vi "Begin.vi"(8 "error in":errorcluster) -> (0 "error out":errorcluster)   [LabVIEW 2016]
doc: "Called before other user functions, this VI is expected to open initial I/O refnums, load in file data, and do all program initialization. Notice that the <B>error out</B> terminal is simply used for data flow. Wiring it to other structures or subVIs ensures that this VI runs first."
uses:
  <vilib>/Rock Robotics/WPI/DriverStation/WPI_DriverStationRobotMode2.ctl
  <vilib>/Rock Robotics/WPI/Joystick/WPI_JoystickDeviceEnum.ctl
  <vilib>/Rock Robotics/WPI/ThirdParty/CanMotor/TalonSRX/WPI_CANTalonSRX_APIControlMode.ctl
  <vilib>/Rock Robotics/WPI/ThirdParty/CanMotor/TalonSRX/WPI_CANTalonSRX_APIFeedbackSelect.ctl
  <vilib>/Rock Robotics/SystemInterfaces/DIO/FPGA_DIOChannel.ctl
  <vilib>/Rock Robotics/SystemInterfaces/spilib/spi_bus.ctl
  <vilib>/Rock Robotics/SystemInterfaces/DIO/FPGA_DIOPWMChannel.ctl
  <vilib>/Rock Robotics/WPI/SafetyOutput/WPI_SafetyOutputConfigMenu.ctl
  Robot Global Data.vi
  <vilib>/Rock Robotics/Network Tables/NT Write String Array.vi
  <vilib>/Rock Robotics/WPI/Counter/WPI_CounterDigitalInputToDigitalSource.vi
  <vilib>/Rock Robotics/WPI/Switch/WPI_SwitchOpenLimit.vi
  <vilib>/Rock Robotics/WPI/Gyro/WPI_GyroAnalogOpen.vi
  <vilib>/Rock Robotics/WPI/RobotDrive/WPI_RobotDriveOpen4MotorWithExistingMotors.vi
  <vilib>/Rock Robotics/WPI/RobotDrive/WPI_RobotDriveOpen4MotorWithTalon.vi
  <vilib>/Rock Robotics/WPI/MotorControl/WPI_MotorControlOpen SPARK.vi
  <vilib>/Rock Robotics/WPI/MotorControl/WPI_MotorControlOpen Victor.vi
  <vilib>/Rock Robotics/WPI/Solenoid/WPI_SolenoidOpenSingle.vi
  <vilib>/Rock Robotics/WPI/Solenoid/WPI_SolenoidChannel.ctl
panel:
  out "error out 2":errorcluster
  in  "Number Encoder Lines\n(Counts Per Rotation)":u32=309
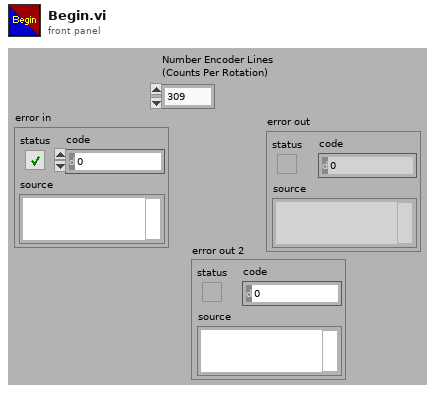
[diagram p1: front panel]
types:
  T1 = typedef "spi_bus.ctl" = enum16{"SPI On-Board, CS0", "SPI On-Board, CS1", "SPI On-Board, CS2", "SPI On-Board, CS3", "SPI MXP", "Invalid"}
  T2 = typedef "FPGA_DIOChannel.ctl" = enum8{"DIO 0", "DIO 1", "DIO 2", "DIO 3", "DIO 4", "DIO 5", "DIO 6", "DIO 7", "DIO 8", "DIO 9", "DIO MXP 0", "DIO MXP 1", "DIO MXP 2", "DIO MXP 3", "DIO MXP 4", "DIO MXP 5", "DIO MXP 6", "DIO MXP 7", "DIO MXP 8", "DIO MXP 9", "DIO MXP 10", "DIO MXP 11", "DIO MXP 12", "DIO MXP 13", "DIO MXP 14", "DIO MXP 15", "SPI Port CS1", "SPI Port CS2", "SPI Port CS3", "SPI Port MISO", "SPI Port MOSI", "Invalid"}
  T3 = typedef "WPI_CANTalonSRX_APIFeedbackSelect.ctl" = enum16{"Digital Quadrature Encoder", "Analog Potentiometer", "Analog Encoder", "Count on Quad-A (Rising-Edge)", "Count on Quad-A (Falling-Edge)", "CTR Magnetic Enc (Absolute)", "CTR Magnetic Enc (Relative)", "Pulse Width"}
  T4 = typedef "WPI_CANTalonSRX_APIControlMode.ctl" = enum8{"Percent VBus", "Speed", "Position", "Slave", "Unchanged / Invalid", "Voltage Compensation", "Current", "Motion Profile", "Motion Magic"}
  T5 = typedef "WPI_JoystickDeviceEnum.ctl" = enum16{"USB 0", "USB 1", "USB 2", "USB 3", "USB 4", "USB 5"}
  T6 = typedef "WPI_DriverStationRobotMode2.ctl" = enum16{"Autonomous Disabled", "Autonomous Enabled", "Teleop Disabled", "Teleop Enabled", "Disconnected", "Finish", "Test Disabled", "Test Enabled", "Emergency Stopped"}
  T7 = typedef "WPI_MotorControlDeviceRef.ctl" = cluster{"DeviceStatus":errorcluster, "Type":T8, "PWM":cluster{"PWM Channel":T9, "DeadBand":T10}, "CAN":cluster{"Device Number":u8, "SetOutput VI Ref":variant, "GetOutput VI Ref":variant, "Enable VI Ref":variant, "Disable VI Ref":variant, "Data":variant}, "Invert":bool}
  T8 = typedef "WPI_MotorControlType.ctl" = enum16{"PWM", "CAN"}
  T9 = typedef "FPGA_DIOPWMChannel.ctl" = enum8{"PWM 0", "PWM 1", "PWM 2", "PWM 3", "PWM 4", "PWM 5", "PWM 6", "PWM 7", "PWM 8", "PWM 9", "PWM MXP 0", "PWM MXP 1", "PWM MXP 2", "PWM MXP 3", "PWM MXP 4", "PWM MXP 5", "PWM MXP 6", "PWM MXP 7", "PWM MXP 8", "PWM MXP 9", "Invalid"}
  T10 = typedef "WPI_PWMDeadband.ctl" = cluster{"Name":string, "maxPositivePwm":i32, "minPositivePwm":i32, "centerPwm":i32, "maxNegativePwm":i32, "minNegativePwm":i32, "angularRange":u16}
  T11 = typedef "WPI_GyroDevRef.ctl" = cluster{"DevStatus":errorcluster, "Analog Channel":T12, "Offset":dbl, "Gain (VoltsPerDegree/Second)":dbl, "Gyro Type":enum16{"Analog", "XRS450"}, "Handle":i32, "SPI Bus":T1, "Device Found":bool, "Sample Rate":dbl, "Calibrate On Open":bool}
  T12 = typedef "FPGA_AIChannel.ctl" = enum8{"AI 0", "AI 1", "AI 2", "AI 3", "AI MXP 0", "AI MXP 1", "AI MXP 2", "AI MXP 3", "Invalid"}
  T13 = typedef "WPI_SafetyOutputConfigMenu.ctl" = enum16{"Enable", "Disable"}
  T14 = typedef "WPI_RobotDriveDevRef.ctl" = cluster{"DevStatus":errorcluster, "Motors[]":T7[], "Square Inputs":bool, "Max Output":dbl}
  T15 = typedef "WPI_ServoDeviceRef.ctl" = cluster{"DeviceStatus":errorcluster, "PWM Channel":T9, "DeadBand":T10}
  T16 = typedef "WPI_JoystickDevRef.ctl" = cluster{"Device":T5}
  T17 = typedef "WPI_SwitchDevRef.ctl" = cluster{"DevStatus":errorcluster, "DIO Channel":T2, "CntIndex":T18, "Normally Closed":bool}
  T18 = typedef "FPGA_CounterCtrSystemIndex.ctl" = enum8{"Ctr 0", "Ctr 1", "Ctr 2", "Ctr 3", "Ctr 4", "Ctr 5", "Ctr 6", "Ctr 7", "Invalid"}
  T19 = typedef "WPI_SolenoidChannel.ctl" = enum8{"Solenoid 0", "Solenoid 1", "Solenoid 2", "Solenoid 3", "Solenoid 4", "Solenoid 5", "Solenoid 6", "Solenoid 7", "Invalid"}
  T20 = typedef "WPI_SolenoidDevRef.ctl" = cluster{"DevStatus":errorcluster, "Pneumatics Control Module":u8, "Forward Solenoid Channel":T19, "Reverse Solenoid Channel":T19}
  T21 = typedef "WPI_DigitalInputDevRef.ctl" = cluster{"DevStatus":errorcluster, "DIO Channel":T2}
  T22 = typedef "FPGA_CounterEncoderSourceConvertionLVSourceType.ctl" = cluster{"DevStatus":errorcluster, "AnalogTriggerMode?":bool, "DigitalMode":cluster{"DIO Channel":T23}, "AnalogTriggerMode":cluster{"AnalogTriggerIndex":T24, "OutputType":T25}}
  T23 = typedef "FPGA_DIODigitalSourceChannel.ctl" = enum8{"DIO 0", "DIO 1", "DIO 2", "DIO 3", "DIO 4", "DIO 5", "DIO 6", "DIO 7", "DIO 8", "DIO 9", "DIO MXP 0", "DIO MXP 1", "DIO MXP 2", "DIO MXP 3", "DIO MXP 4", "DIO MXP 5", "DIO MXP 6", "DIO MXP 7", "DIO MXP 8", "DIO MXP 9", "DIO MXP 10", "DIO MXP 11", "DIO MXP 12", "DIO MXP 13", "DIO MXP 14", "DIO MXP 15", "Disabled"}
  T24 = typedef "FPGA_AnalogTriggerIndex.ctl" = enum8{"Trig 0", "Trig 1", "Trig 2", "Trig 3", "Trig 4", "Trig 5", "Trig 6", "Trig 7", "Invalid"}
  T25 = typedef "FPGA_AnalogTriggerOutType.ctl" = enum16{"InWindow", "TriggerState", "Rising", "Falling"}
  T26 = typedef "WPI_EncoderDevRef.ctl" = cluster{"DevStatus":errorcluster, "EncoderIndex":T27, "CounterIndex":T18, "DistancePerCount":dbl, "Decoding Type":T28}
  T27 = typedef "FPGA_EncoderIdx.ctl" = enum8{"Enc 0", "Enc 1", "Enc 2", "Enc 3", "Enc 4", "Enc 5", "Enc 6", "Enc 7", "Invalid"}
  T28 = typedef "WPI_EncoderType.ctl" = enum16{"1x", "2x", "4x"}
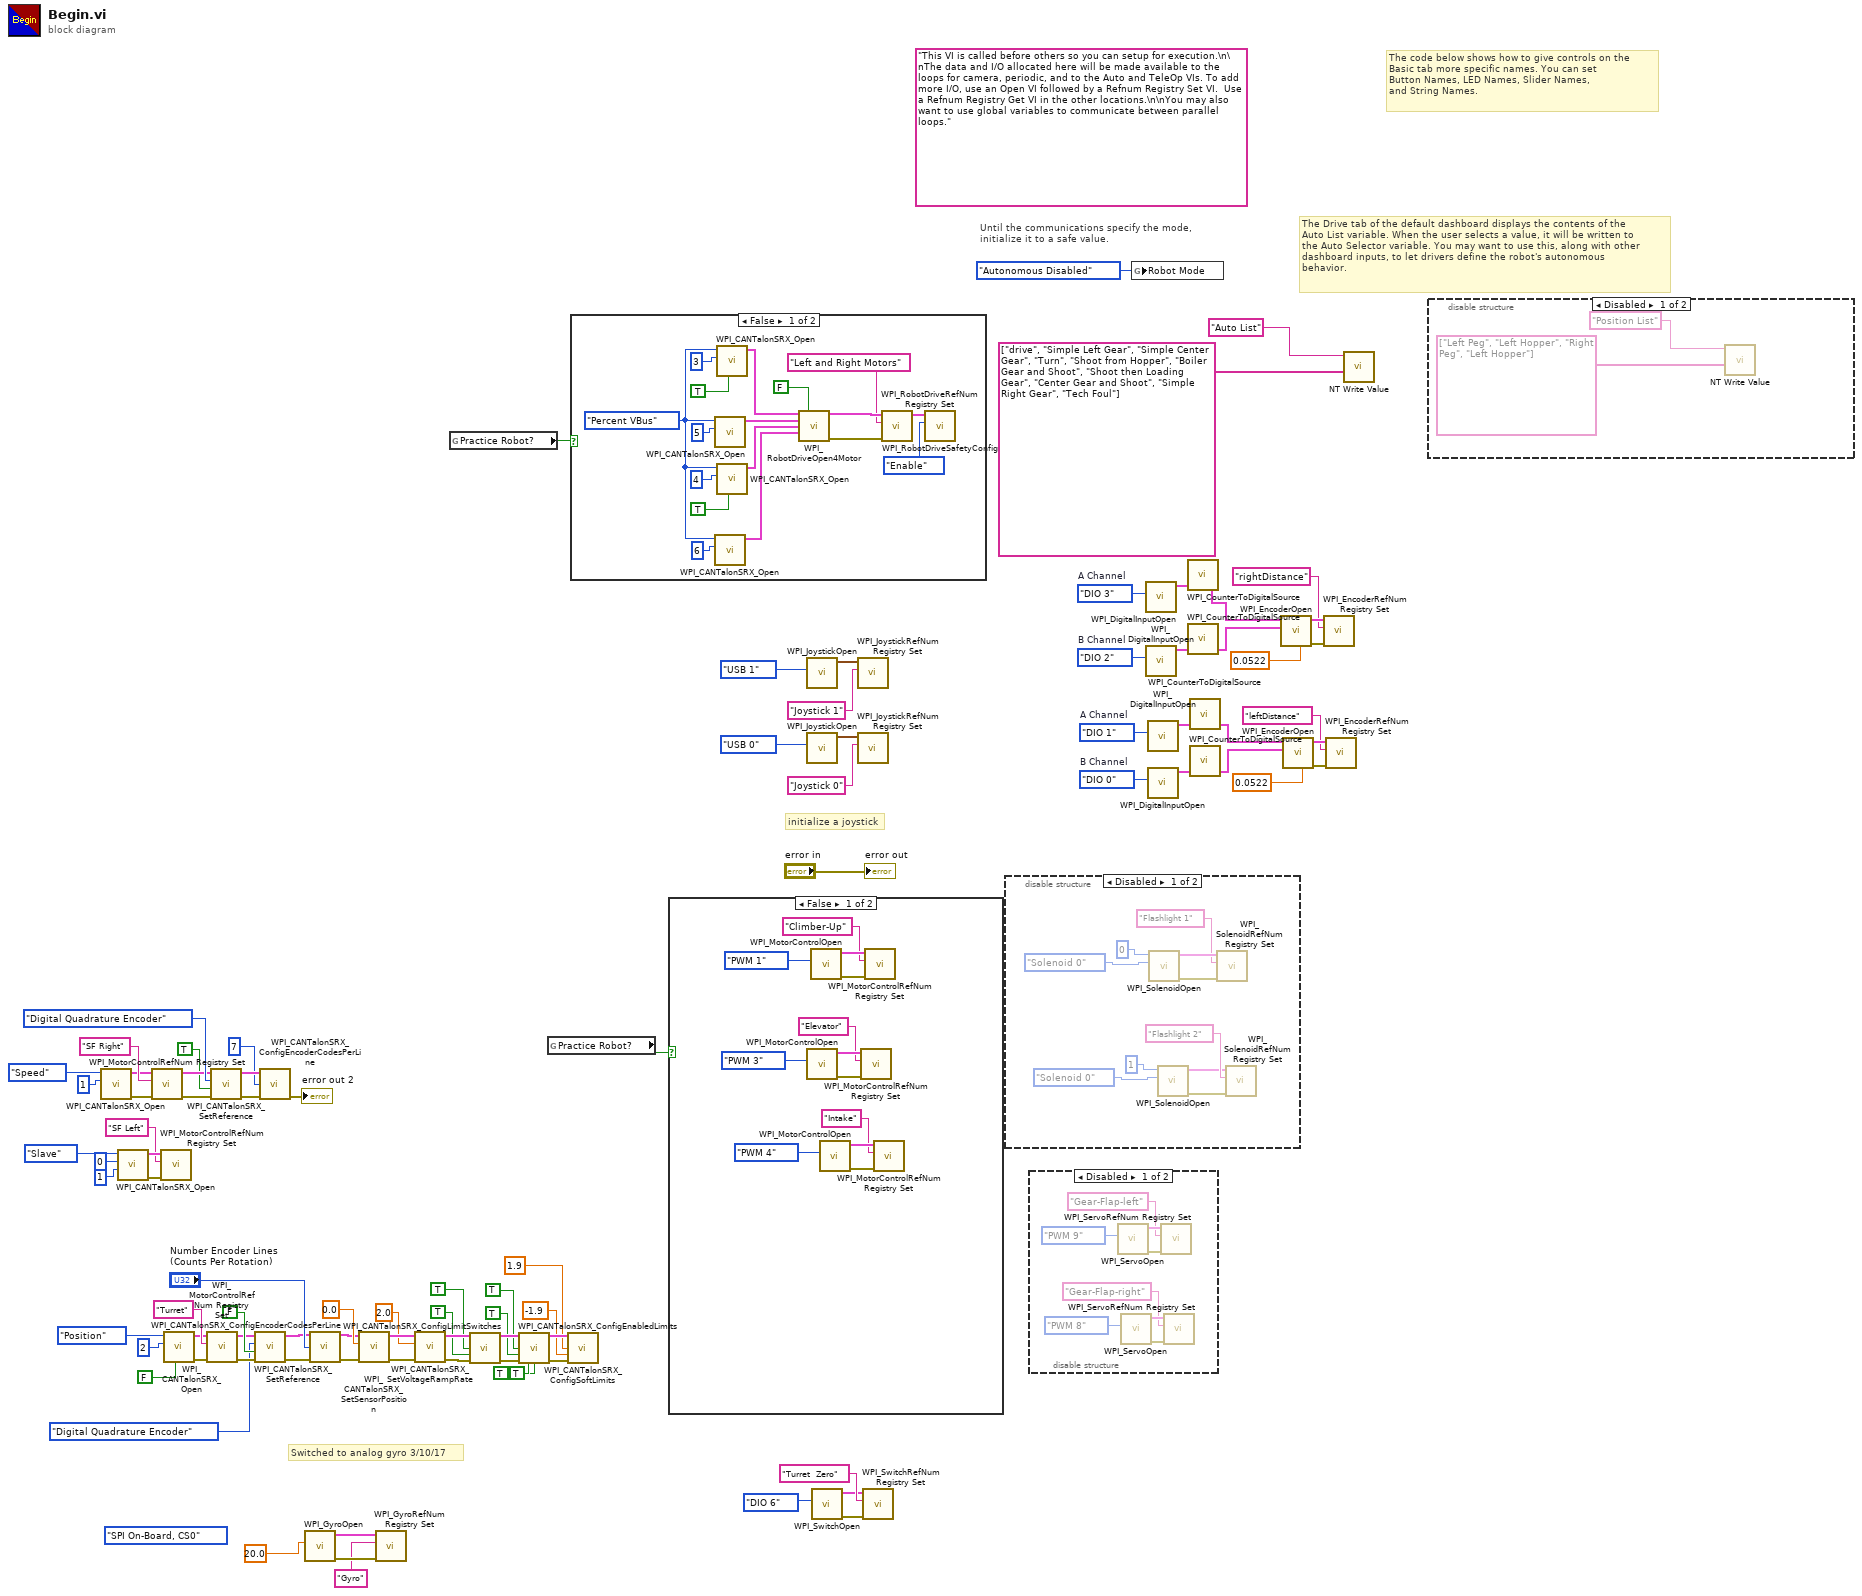
[diagram p0: block diagram]
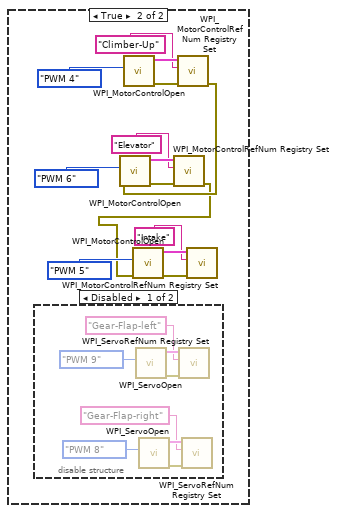
[diagram p5: hidden frame]
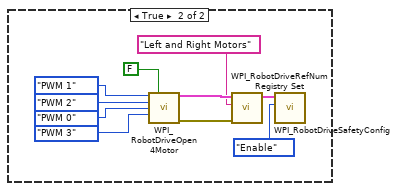
[diagram p7: hidden frame]
diagram:
  (unwired) spi_bus."SPI On-Board, CS0" ("SPI Bus")
  w38 = FPGA_DIOChannel."DIO 2"  # B Channel
  w37 = FPGA_DIOChannel."DIO 3"  # A Channel
  w47 = FPGA_DIOChannel."DIO 0"  # B Channel
  w46 = FPGA_DIOChannel."DIO 1"  # A Channel
  (unwired) "This VI is called before others so you can setup for execution.\n\nThe data and I/O allocated here will be made available to the loops for camera, periodic, and to the Auto and TeleOp VIs. To add more I/O, use an Open VI followed by a Refnum Registry Set VI.  Use a Refnum Registry Get VI in the other locations.\n\nYou may also want to use global variables to communicate between parallel loops."
  # "Switched to analog gyro 3/10/17"
  # "The Drive tab of the default dashboard displays the contents of the\nAuto List variable. When the user selects a value, it will be written to\nthe Auto Selector variable. You may want to use this, along with other\ndashboard inputs, to let drivers define the robot's autonomous\nbehavior."
  # "The code below shows how to give controls on the\nBasic tab more specific names. You can set\nButton Names, LED Names, Slider Names,\nand String Names."
  # "initialize a joystick"
  # "Until the communications specify the mode,\ninitialize it to a safe value."
  n1 = call <vilib>:"WPI_CANTalonSRX_Open.vi"("Device Number"=u8 1, "Control Mode"=WPI_CANTalonSRX_APIControlMode."Speed") -> ("error out"=w68:errorcluster, "CAN Talon SRX Ref"=w67:T7)  [unwired: 8 in]
  n2 = call <vilib>:"WPI_CANTalonSRX_Open.vi"("Master Device Number"=u8 1, "Device Number"=u8 0, "Control Mode"=WPI_CANTalonSRX_APIControlMode."Slave") -> ("error out"=w75:errorcluster, "CAN Talon SRX Ref"=w76:T7)  [unwired: 7 in]
  n3 = call <vilib>:"WPI_MotorControlRefNum Registry Set.vi"("error in (no error)"=w68, "refnum name"="SF Right", "MotorControlDevRef"=w67) -> ("error out"=w49:errorcluster, "MotorControlDevRef"=w50:T7)  [unwired: 7 in]
  n4 = call <vilib>:"WPI_MotorControlRefNum Registry Set.vi"("error in (no error)"=w75, "refnum name"="SF Left", "MotorControlDevRef"=w76) -> ()  [unwired: 7 in, 2 out]
  n5 = call <vilib>:"WPI_CANTalonSRX_Open.vi"("Invert"=FALSE, "Device Number"=u8 2, "Control Mode"=WPI_CANTalonSRX_APIControlMode."Position") -> ("error out"=w59:errorcluster, "CAN Talon SRX Ref"=w61:T7)  [unwired: 7 in]
  n6 = call <vilib>:"WPI_MotorControlRefNum Registry Set.vi"("error in (no error)"=w59, "refnum name"="Turret", "MotorControlDevRef"=w61) -> ("error out"=w58:errorcluster, "MotorControlDevRef"=w60:T7)  [unwired: 7 in]
  n7 = call <vilib>:"WPI_CANTalonSRX_SetReference.vi"("error in (no error)"=w49, "Reverse Feedback Sensor"=TRUE, "Feedback Reference"=WPI_CANTalonSRX_APIFeedbackSelect."Digital Quadrature Encoder", "CAN Talon SRX Ref"=w50) -> ("error out"=w48:errorcluster, "CAN Talon SRX Ref"=w53:T7)  [unwired: 6 in]
  n8 = call <vilib>:"WPI_CANTalonSRX_SetReference.vi"("error in (no error)"=w58, "Reverse Feedback Sensor"=FALSE, "Feedback Reference"=WPI_CANTalonSRX_APIFeedbackSelect."Digital Quadrature Encoder", "CAN Talon SRX Ref"=w60) -> ("error out"=w57:errorcluster, "CAN Talon SRX Ref"=w63:T7)  [unwired: 6 in]
  n9 = call <vilib>:"WPI_CANTalonSRX_ConfigEncoderCodesPerLine.vi"("CAN Talon SRX Ref"=w53, "Number Encoder Lines\n(Counts Per Rotation)"=u32 7 ("Number Encoder Lines\n(Counts Per Rotation)"), "error in (no error)"=w48) -> ("error out"=→"error out 2":errorcluster)  [unwired: 11 in, 1 out]
  n10 = call-poly <vilib>:"WPI_GyroOpen.vi"("Analog Channel"=20.0 ("Calibration Time (s)")) -> ("error out"=w20:errorcluster, "GyroDevRef"=w19:T11)  [unwired: 8 in, 1 out]
  n11 = call <vilib>:"WPI_CANTalonSRX_ConfigEncoderCodesPerLine.vi"("CAN Talon SRX Ref"=w63, "Number Encoder Lines\n(Counts Per Rotation)"="Number Encoder Lines\n(Counts Per Rotation)", "error in (no error)"=w57) -> ("CAN Talon SRX Ref"=w55:T7, "error out"=w56:errorcluster)  [unwired: 11 in]
  n12 = call <vilib>:"WPI_CANTalonSRX_SetSensorPosition.vi"("error in (no error)"=w56, "New Sensor Position"=0.0, "CAN Talon SRX Ref"=w55) -> ("error out"=w23:errorcluster, "CAN Talon SRX Ref"=w22:T7)  [unwired: 7 in]
  n13 = call <vilib>:"WPI_GyroRefNum Registry Set.vi"("error in (no error)"=w20, "refnum name"="Gyro", "GyroDevRef"=w19) -> ()  [unwired: 7 in, 2 out]
  n14 = call <vilib>:"WPI_CANTalonSRX_SetVoltageRampRate.vi"("error in (no error)"=w23, "Throttle Ramp Rate (percent/s)"=2.0, "CAN Talon SRX Ref"=w22) -> ("error out"=w13:errorcluster, "CAN Talon SRX Ref"=w14:T7)  [unwired: 7 in]
  n15 = global read "Robot Global Data.vi" "Practice Robot?"() -> (w82:bool)
  n16 = call <vilib>:"WPI_CANTalonSRX_ConfigLimitSwitches.vi"("CAN Talon SRX Ref"=w14, "Forward Limit Switch Normally Open"=TRUE, "Reverse Limit Switch Normally Open"=TRUE, "error in (no error)"=w13) -> ("CAN Talon SRX Ref"=w10:T7, "error out"=w9:errorcluster)  [unwired: 10 in]
  n17 = call <vilib>:"WPI_CANTalonSRX_ConfigEnabledLimits.vi"("CAN Talon SRX Ref"=w10, "Forward Limit Switch Enable"=TRUE, "Reverse Limit Switch Enable"=TRUE, "error in (no error)"=w9, "Forward Soft Limit Enable"=TRUE, "Reverse Soft Limit Enable"=TRUE) -> ("CAN Talon SRX Ref"=w6:T7, "error out"=w5:errorcluster)  [unwired: 8 in]
  n18 = global read "Robot Global Data.vi" "Practice Robot?"() -> (w81:bool)
  n19 = call <vilib>:"WPI_CANTalonSRX_ConfigSoftLimits.vi"("CAN Talon SRX Ref"=w6, "Forward Limit Position"=1.9 ("Upper Limit Position"), "Reverse Limit Position"=-1.9 ("Lower Limit Position"), "error in (no error)"=w5) -> ()  [unwired: 10 in, 2 out]
  n20 = case shown="False" w82 {
    frame False {
      w100 = WPI_CANTalonSRX_APIControlMode."Percent VBus" ("Control Mode")
      n21 = call <vilib>:"WPI_CANTalonSRX_Open.vi"("Device Number"=u8 5, "Control Mode"=w100) -> ("CAN Talon SRX Ref"=w103:T7)  [unwired: 8 in, 1 out]
      n22 = call <vilib>:"WPI_CANTalonSRX_Open.vi"("Device Number"=u8 6, "Control Mode"=w100) -> ("CAN Talon SRX Ref"=w101:T7)  [unwired: 8 in, 1 out]
      n23 = call <vilib>:"WPI_CANTalonSRX_Open.vi"("Invert"=TRUE, "Device Number"=u8 3, "Control Mode"=w100) -> ("CAN Talon SRX Ref"=w104:T7)  [unwired: 7 in, 1 out]
      n24 = call <vilib>:"WPI_CANTalonSRX_Open.vi"("Invert"=TRUE, "Device Number"=u8 4, "Control Mode"=w100) -> ("CAN Talon SRX Ref"=w102:T7)  [unwired: 7 in, 1 out]
      n25 = call-poly <vilib>:"WPI_RobotDriveOpen4Motor.vi"("Rear Left Motor Dev Ref"=w104, "Square Inputs"=FALSE, "Rear Right Motor Dev Ref"=w103, "Front Left Motor Dev Ref"=w102, "Front Right Motor Dev Ref"=w101) -> ("RobotDriveDevRef"=w109:T14, "error out"=w107:errorcluster)  [unwired: 9 in]
      n26 = call <vilib>:"WPI_RobotDriveRefNum Registry Set.vi"("error in (no error)"=w107, "refnum name"="Left and Right Motors", "RobotDriveDevRef"=w109) -> ("RobotDriveDevRef"=w106:T14)  [unwired: 1 in, 7 out]
      n27 = call <vilib>:"WPI_RobotDriveSafetyConfig.vi"("mode"=WPI_SafetyOutputConfigMenu."Enable", "RobotDriveDevRef"=w106) -> ()  [unwired: 8 in, 2 out]
    }
    frame True {
      n28 = call-poly <vilib>:"WPI_RobotDriveOpen4Motor.vi"("Rear Left Motor"=FPGA_DIOPWMChannel."PWM 1", "Rear Left Motor Inverted"=FALSE ("Square Inputs"), "Rear Right Motor"=FPGA_DIOPWMChannel."PWM 2", "Front Left Motor"=FPGA_DIOPWMChannel."PWM 0", "Front Right Motor"=FPGA_DIOPWMChannel."PWM 3") -> ("RobotDriveDevRef"=w119:T14, "error out"=w117:errorcluster)  [unwired: 9 in]
      n29 = call <vilib>:"WPI_RobotDriveRefNum Registry Set.vi"("error in (no error)"=w117, "refnum name"="Left and Right Motors", "RobotDriveDevRef"=w119) -> ("RobotDriveDevRef"=w116:T14)  [unwired: 1 in, 7 out]
      n30 = call <vilib>:"WPI_RobotDriveSafetyConfig.vi"("mode"=WPI_SafetyOutputConfigMenu."Enable", "RobotDriveDevRef"=w116) -> ()  [unwired: 8 in, 2 out]
    }
  }
  n31 = case shown="False" w81 {
    frame False {
      n32 = call-poly <vilib>:"WPI_MotorControlOpen.vi"("PWM Channel"=FPGA_DIOPWMChannel."PWM 3") -> ("error out"=w131:errorcluster, "MotorControlDeviceRef"=w130:T7)  [unwired: 9 in]
      n33 = call-poly <vilib>:"WPI_MotorControlOpen.vi"("PWM Channel"=FPGA_DIOPWMChannel."PWM 1") -> ("error out"=w127:errorcluster, "MotorControlDeviceRef"=w126:T7)  [unwired: 9 in]
      n34 = call-poly <vilib>:"WPI_MotorControlOpen.vi"("PWM Channel"=FPGA_DIOPWMChannel."PWM 4") -> ("error out"=w123:errorcluster, "MotorControlDeviceRef"=w122:T7)  [unwired: 9 in]
      n35 = call <vilib>:"WPI_MotorControlRefNum Registry Set.vi"("error in (no error)"=w131, "refnum name"="Elevator", "MotorControlDevRef"=w130) -> ()  [unwired: 7 in, 2 out]
      n36 = call <vilib>:"WPI_MotorControlRefNum Registry Set.vi"("error in (no error)"=w127, "refnum name"="Climber-Up", "MotorControlDevRef"=w126) -> ()  [unwired: 7 in, 2 out]
      n37 = call <vilib>:"WPI_MotorControlRefNum Registry Set.vi"("error in (no error)"=w123, "refnum name"="Intake", "MotorControlDevRef"=w122) -> ()  [unwired: 7 in, 2 out]
    }
    frame True {
      n38 = disable-structure shown="Disabled" {
        frame Disabled {
          n39 = call <vilib>:"WPI_ServoOpen.vi"("PWM Channel"=FPGA_DIOPWMChannel."PWM 9") -> ("error out"=w148:errorcluster, "ServoDeviceRef"=w153:T15)  [unwired: 9 in]
          n40 = call <vilib>:"WPI_ServoOpen.vi"("PWM Channel"=FPGA_DIOPWMChannel."PWM 8") -> ("error out"=w149:errorcluster, "ServoDeviceRef"=w152:T15)  [unwired: 9 in]
          n41 = call <vilib>:"WPI_ServoRefNum Registry Set.vi"("error in (no error)"=w148, "refnum name"="Gear-Flap-left", "ServoDeviceRef"=w153) -> ()  [unwired: 7 in, 2 out]
          n42 = call <vilib>:"WPI_ServoRefNum Registry Set.vi"("error in (no error)"=w149, "refnum name"="Gear-Flap-right", "ServoDeviceRef"=w152) -> ()  [unwired: 7 in, 2 out]
        }
        frame Enabled {
        }
      }
      n43 = call-poly <vilib>:"WPI_MotorControlOpen.vi"("PWM Channel"=FPGA_DIOPWMChannel."PWM 4") -> ("error out"=w141:errorcluster, "MotorControlDeviceRef"=w140:T7)  [unwired: 9 in]
      n44 = call <vilib>:"WPI_MotorControlRefNum Registry Set.vi"("error in (no error)"=w141, "refnum name"="Climber-Up", "MotorControlDevRef"=w140) -> ("error out"=w133:errorcluster)  [unwired: 7 in, 1 out]
      n45 = call-poly <vilib>:"WPI_MotorControlOpen.vi"("error in (no error)"=w133, "PWM Channel"=FPGA_DIOPWMChannel."PWM 6") -> ("error out"=w145:errorcluster, "MotorControlDeviceRef"=w144:T7)  [unwired: 8 in]
      n46 = call <vilib>:"WPI_MotorControlRefNum Registry Set.vi"("error in (no error)"=w145, "refnum name"="Elevator", "MotorControlDevRef"=w144) -> ("error out"=w132:errorcluster)  [unwired: 7 in, 1 out]
      n47 = call-poly <vilib>:"WPI_MotorControlOpen.vi"("error in (no error)"=w132, "PWM Channel"=FPGA_DIOPWMChannel."PWM 5") -> ("error out"=w137:errorcluster, "MotorControlDeviceRef"=w136:T7)  [unwired: 8 in]
      n48 = call <vilib>:"WPI_MotorControlRefNum Registry Set.vi"("error in (no error)"=w137, "refnum name"="Intake", "MotorControlDevRef"=w136) -> ()  [unwired: 7 in, 2 out]
    }
  }
  n49 = call <vilib>:"WPI_JoystickOpen.vi"("JoystickDevice"=WPI_JoystickDeviceEnum."USB 1") -> ("JoystickDevRef"=w85:T16)  [unwired: 10 in]
  n50 = call <vilib>:"WPI_JoystickOpen.vi"("JoystickDevice"=WPI_JoystickDeviceEnum."USB 0") -> ("JoystickDevRef"=w90:T16)  [unwired: 10 in]
  n51 = call-poly <vilib>:"WPI_SwitchOpen.vi"("DIO Channel"=FPGA_DIOChannel."DIO 6") -> ("error out"=w25:errorcluster, "SwitchDevRef"=w26:T17)  [unwired: 9 in]
  n52 = call <vilib>:"WPI_JoystickRefNum Registry Set.vi"("refnum name"="Joystick 1", "JoystickDevRef"=w85) -> ()  [unwired: 8 in, 2 out]
  n53 = call <vilib>:"WPI_JoystickRefNum Registry Set.vi"("refnum name"="Joystick 0", "JoystickDevRef"=w90) -> ()  [unwired: 8 in, 2 out]
  n54 = call <vilib>:"WPI_SwitchRefNum Registry Set.vi"("error in (no error)"=w25, "refnum name"="Turret  Zero", "SwitchDevRef"=w26) -> ()  [unwired: 7 in, 2 out]
  n55 = disable-structure shown="Disabled" {
    frame Disabled {
      n56 = call-poly <vilib>:"WPI_SolenoidOpen.vi"("Solenoid Channel"=WPI_SolenoidChannel."Solenoid 0", "Pneumatics Control Module (0)"=u8 0) -> ("error out"=w161:errorcluster, "SolenoidDevRef"=w160:T20)  [unwired: 8 in]
      n57 = call-poly <vilib>:"WPI_SolenoidOpen.vi"("Solenoid Channel"=WPI_SolenoidChannel."Solenoid 0", "Pneumatics Control Module (0)"=u8 1) -> ("error out"=w156:errorcluster, "SolenoidDevRef"=w157:T20)  [unwired: 8 in]
      n58 = call <vilib>:"WPI_SolenoidRefNum Registry Set.vi"("error in (no error)"=w161, "refnum name"="Flashlight 1", "SolenoidDevRef"=w160) -> ()  [unwired: 7 in, 2 out]
      n59 = call <vilib>:"WPI_SolenoidRefNum Registry Set.vi"("error in (no error)"=w156, "refnum name"="Flashlight 2", "SolenoidDevRef"=w157) -> ()  [unwired: 7 in, 2 out]
    }
    frame Enabled {
    }
  }
  n60 = disable-structure shown="Disabled" {
    frame Disabled {
      n61 = call <vilib>:"WPI_ServoOpen.vi"("PWM Channel"=FPGA_DIOPWMChannel."PWM 9") -> ("error out"=w166:errorcluster, "ServoDeviceRef"=w171:T15)  [unwired: 9 in]
      n62 = call <vilib>:"WPI_ServoOpen.vi"("PWM Channel"=FPGA_DIOPWMChannel."PWM 8") -> ("error out"=w167:errorcluster, "ServoDeviceRef"=w170:T15)  [unwired: 9 in]
      n63 = call <vilib>:"WPI_ServoRefNum Registry Set.vi"("error in (no error)"=w166, "refnum name"="Gear-Flap-left", "ServoDeviceRef"=w171) -> ()  [unwired: 7 in, 2 out]
      n64 = call <vilib>:"WPI_ServoRefNum Registry Set.vi"("error in (no error)"=w167, "refnum name"="Gear-Flap-right", "ServoDeviceRef"=w170) -> ()  [unwired: 7 in, 2 out]
    }
    frame Enabled {
    }
  }
  n65 = global write "Robot Global Data.vi" "Robot Mode"(WPI_DriverStationRobotMode2."Autonomous Disabled" ("Robot Mode")) -> ()
  n66 = call <vilib>:"WPI_DigitalInputOpen.vi"("DIO Channel"=w37) -> ("DigitalInputDevRef"=w34:T21)  [unwired: 1 in, 9 out]
  n67 = call <vilib>:"WPI_DigitalInputOpen.vi"("DIO Channel"=w38) -> ("DigitalInputDevRef"=w35:T21)  [unwired: 1 in, 9 out]
  n68 = call <vilib>:"WPI_DigitalInputOpen.vi"("DIO Channel"=w46) -> ("DigitalInputDevRef"=w43:T21)  [unwired: 1 in, 9 out]
  n69 = call <vilib>:"WPI_DigitalInputOpen.vi"("DIO Channel"=w47) -> ("DigitalInputDevRef"=w44:T21)  [unwired: 1 in, 9 out]
  n70 = call-poly <vilib>:"WPI_CounterToDigitalSource.vi"("DigitalInputDevRef"=w34) -> ("Digital Source"=w33:T22)  [unwired: 6 out]
  n71 = call-poly <vilib>:"WPI_CounterToDigitalSource.vi"("DigitalInputDevRef"=w35) -> ("Digital Source"=w36:T22)  [unwired: 6 out]
  n72 = call-poly <vilib>:"WPI_CounterToDigitalSource.vi"("DigitalInputDevRef"=w43) -> ("Digital Source"=w42:T22)  [unwired: 6 out]
  n73 = call-poly <vilib>:"WPI_CounterToDigitalSource.vi"("DigitalInputDevRef"=w44) -> ("Digital Source"=w45:T22)  [unwired: 6 out]
  n74 = call <vilib>:"WPI_EncoderOpen.vi"("DistancePerCount"=0.0522, "BSource"=w36, "ASource"=w33) -> ("error out"=w32:errorcluster, "EncoderDevRef"=w31:T26)  [unwired: 5 in, 2 out]
  n75 = call <vilib>:"WPI_EncoderOpen.vi"("DistancePerCount"=0.0522, "BSource"=w45, "ASource"=w42) -> ("error out"=w41:errorcluster, "EncoderDevRef"=w40:T26)  [unwired: 5 in, 2 out]
  n76 = call <vilib>:"WPI_EncoderRefNum Registry Set.vi"("error in (no error)"=w32, "refnum name"="rightDistance", "EncoderDevRef"=w31) -> ()  [unwired: 7 in, 2 out]
  n77 = call <vilib>:"WPI_EncoderRefNum Registry Set.vi"("error in (no error)"=w41, "refnum name"="leftDistance", "EncoderDevRef"=w40) -> ()  [unwired: 7 in, 2 out]
  n78 = call-poly <vilib>:"NT Write Value.vi"("String Array"=string[] ["drive", "Simple Left Gear", "Simple Center Gear", "Turn", "Shoot from Hopper", "Boiler Gear and Shoot", "Shoot then Loading Gear", "Center Gear and Shoot", "Simple Right Gear", "Tech Foul"], "Name"="Auto List") -> ()  [unwired: 9 in, 1 out]
  n79 = disable-structure shown="Disabled" {
    frame Disabled {
      n80 = call-poly <vilib>:"NT Write Value.vi"("String Array"=string[] ["Left Peg", "Left Hopper", "Right Peg", "Left Hopper"], "Name"="Position List") -> ()  [unwired: 9 in, 1 out]
    }
    frame Enabled {
    }
  }
  "error out" <- "error in"
